vi "Relay Auto Tune.VI"(4 "calculate":bool, 5 "autotuning parameters":T3={"Controller Type"=0, "# of cycles to avg"=3, "Relay amplitude (%)"=0.0, "Control design  "=0, "Noise level %"=0.25} {"Noise level %" format="%.2f"; "Control design" items=["Normal", "Fast", "Slow"]; "Relay amplitude (%)" format="%.2f"; "Controller Type" items=["PID", "PI", "P"]}, 6 "options":T2={"sp low"=0.0, "sp high"=100.0, "out low"=-100.0, "out high"=100.0, "hold (F)"=FALSE, "auto (T)"=TRUE, "pro. band (F)"=FALSE, "reverse acting (T)"=TRUE, "beta"=1.0, "linearity"=1.0, "dt (s)"=-1.0} {"dt (s)" format="%.2f"; "linearity" min=0.0 max=1.0 format="%.2f"; "sp low" format="%.2f"; "sp high" format="%.2f"; "out low" format="%.2f"; "out high" format="%.2f"; "beta" min=0.0 max=1.0 format="%.2f"}, 7 "Prev. control out":dbl format="%.2f", 8 "Gain Scheduling Variable":dbl format="%.2f", 9 "gain scheduling":T1={"gain schedule"=[100.0], "PID parameters"=[{"Kc"=4.851751673610237, "Ti (min)"=0.021111111111111112, "Td (min)"=0.005277777777777778}], "scheduling input"=0} {"scheduling input" items=["Set-point", "Process variable", "Controller output", "Gain scheduling input"]; "PID parameters"."Td (min)" format="%.4f"; "PID parameters"."Ti (min)" format="%.4f"; "PID parameters"."Kc" format="%.4f"; "gain schedule" format="%.2f"}, 10 "PV%":dbl(slide)=19.583333333333336 scale=0.0..100.0 scale format="%.1f", 11 "setpoint (%)":dbl(slide)=30.8641975308642 scale=0.0..100.0 scale format="%.1f") -> (0 "setpoint relay":dbl(slide)=30.8641975308642 scale=0.0..100.0 scale format="%.1f", 1 "tuning status":bool, 2 "Tuned PID Parameters":T4 {"Ti" format="%.2f"; "Td" format="%.2f"})   [LabVIEW 2020, in "NI_PID__autopid compat.lvlib"]
doc: "This VI performs the setpoint relay experiment for the autotuning procedure."
uses:
  <vilib>/addons/control/pid/NI_PID__autopid compat.lvlib
  <vilib>/Analysis/baseanly.llb/Mean (DBL).vi
  <vilib>/Analysis/NI_AALBase.lvlib
panel:
  # "Relay Auto Tune"
  # "SP & PV range:"
  # "Output range:"
  # "-1: default,using\nsystem clock"
  # "Prop Band (%)"
  # "Reset Time (min)"
  # "Deriv Time (min)"
  # "Index"
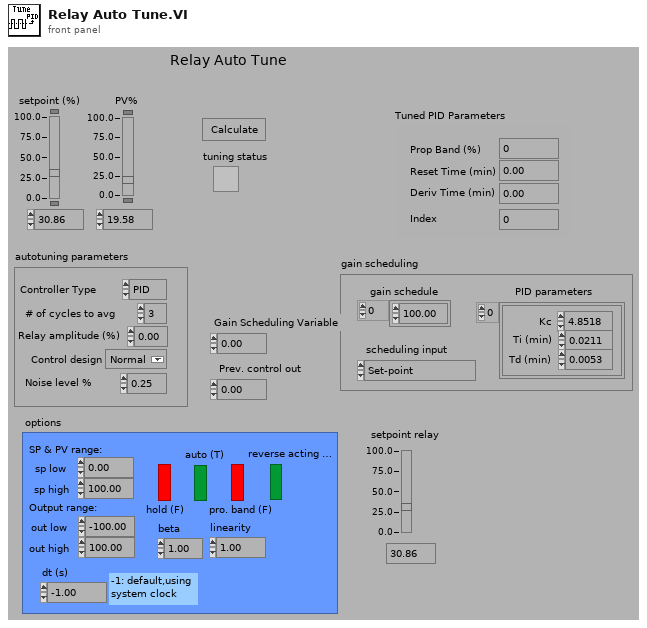
[diagram p1: front panel]
types:
  T1 = cluster{"gain schedule":dbl[], "PID parameters":cluster{"Kc":dbl, "Ti (min)":dbl, "Td (min)":dbl}[], "scheduling input":u16}
  T2 = cluster{"sp low":dbl, "sp high":dbl, "out low":dbl, "out high":dbl, "hold (F)":bool, "auto (T)":bool, "pro. band (F)":bool, "reverse acting (T)":bool, "beta":dbl, "linearity":dbl, "dt (s)":dbl}
  T3 = cluster{"Controller Type":u16, "# of cycles to avg":i32, "Relay amplitude (%)":dbl, "Control design  ":u16, "Noise level %":dbl}
  T4 = cluster{"Kc":dbl, "Ti":dbl, "Td":dbl, "Index":i32}
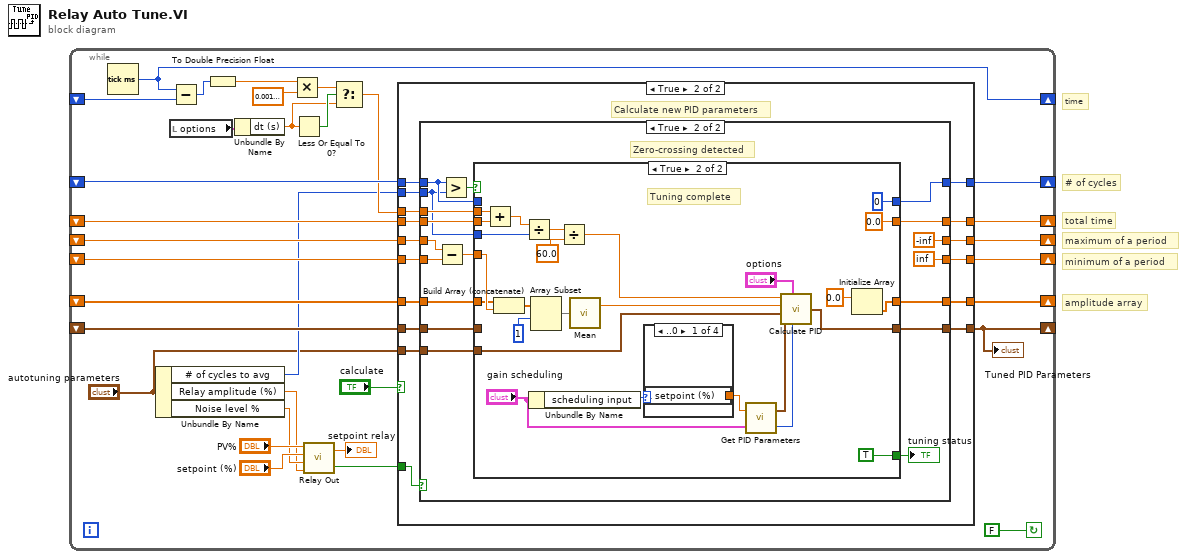
[diagram p0: block diagram]
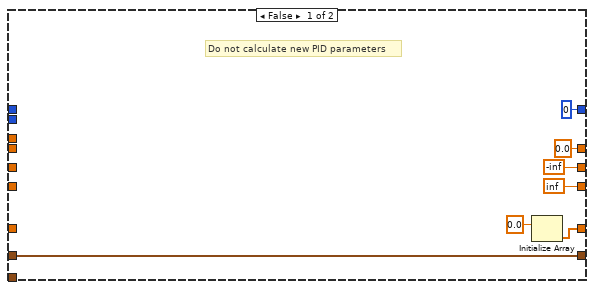
[diagram p2: hidden frame]
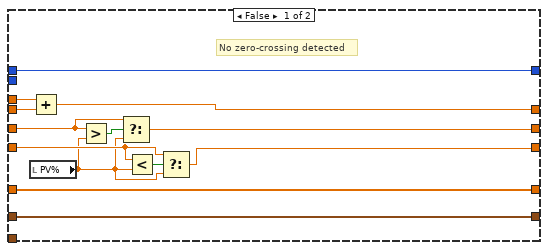
[diagram p3: hidden frame]
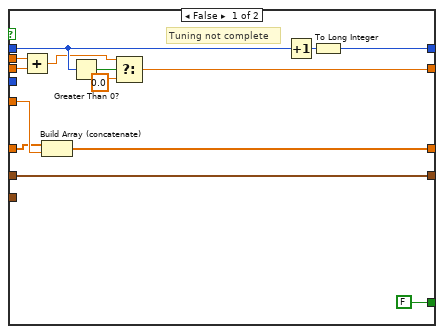
[diagram p4: hidden frame]
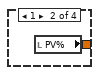
[diagram p5: hidden frame]
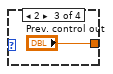
[diagram p6: hidden frame]
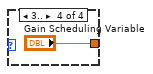
[diagram p7: hidden frame]
diagram:
  # "time"
  # "amplitude array"
  # "total time"
  # "minimum of a period"
  # "maximum of a period"
  # "# of cycles"
  n1 = while {
    shift-left: _ -> [w7]
    shift-right: [w6] -> _
    shift-left: _ -> [w12]
    shift-right: [w13] -> _
    shift-left: _ -> [w23]
    shift-right: [w20] -> _
    shift-left: _ -> [w27]
    shift-right: [w28] -> _
    shift-left: _ -> [w26]
    shift-right: [w29] -> _
    shift-left: _ -> [w30]
    shift-right: [w31] -> _
    shift-left: _ -> [w25]
    shift-right: [w32] -> _
    stop <- FALSE continue-if-true
    n2 = Tick Count (ms)() -> (millisecond timer value=w13:u32)
    n3 = Unbundle By Name("autotuning parameters") -> ("# of cycles to avg"=w3:i32, "Relay amplitude (%)"=w4:dbl, "Noise level %"=w5:dbl)
    n4 = local read "options"() -> (w10:T2)
    n5 = Subtract(x=w13, y=w12) -> (x-y=w16:u32)
    n6 = To Double Precision Float(number=w16) -> (double precision float=w17:dbl)
    n7 = Unbundle By Name(w10) -> ("dt (s)"=w14:dbl)
    n8 = Multiply(x=w17, y=0.0010000000474974513) -> (x*y=w18:dbl)
    n9 = Less Or Equal To 0?(x=w14) -> (x <= 0?=w19:bool)
    n10 = call <vilib>:"Relay Out.vi"("Relay Amp (%)"=w4, "noise disturbance %"=w5, "setpoint %"="setpoint (%)", "PV %"="PV%") -> ("Zero Crossing"=w22:bool, "relay output"=→"setpoint relay":dbl)
    n11 = Select(t=w18, s=w19, f=w14) -> (s? t:f=w11:dbl)
    n12 = case shown="True" "calculate" {
      tunnel: w25 -> [_ w43]
      tunnel: [0 w44] -> w32
      tunnel: [-inf w45] -> w31
      tunnel: w30 -> [_ w55]
      tunnel: w26 -> [_ w54]
      tunnel: [w33 w47] -> w29
      tunnel: [inf w46] -> w28
      tunnel: w27 -> [_ w48]
      tunnel: w3 -> [_ w52]
      tunnel: [w39 w49] -> w20
      tunnel: w23 -> [w39 w53]
      tunnel: w22 -> [_ w51]
      tunnel: w11 -> [_ w50]
      tunnel: w7 -> [_ w42]
      tunnel: [0.0 ("f") w41] -> w6
      tunnel: "autotuning parameters" -> [_ w40]
      frame False {
        # "Do not calculate new PID parameters"
        n13 = Initialize Array(0.0) -> (w33:dbl[])  [unwired: 1 out]
      }
      frame True {
        # "Calculate new PID parameters"
        n14 = case shown="True" w51 {
          tunnel: w43 -> [w68 w73]
          tunnel: [w68 w75] -> w44
          tunnel: [w67 -inf] -> w45
          tunnel: w55 -> [w66 w86]
          tunnel: w54 -> [w65 w84]
          tunnel: [w65 w82] -> w47
          tunnel: [w62 inf] -> w46
          tunnel: w48 -> [w63 w85]
          tunnel: w52 -> [_ w70]
          tunnel: w53 -> [w59 w81]
          tunnel: w50 -> [w57 w80]
          tunnel: [w59 w79] -> w49
          tunnel: w42 -> [w58 w72]
          tunnel: [w56 w71] -> w41
          tunnel: w40 -> [_ w69]
          frame False {
            # "No zero-crossing detected"
            n15 = local read "PV%"() -> (w60:dbl)
            n16 = Add(x=w57, y=w58) -> (x+y=w56:dbl)
            n17 = Greater?(x=w66, y=w60) -> (0:w61:bool)
            n18 = Select(t=w66, s=w61, f=w60) -> (s? t:f=w67:dbl)
            n19 = Less?(x=w63, y=w60) -> (x < y?=w64:bool)
            n20 = Select(t=w63, s=w64, f=w60) -> (s? t:f=w62:dbl)
          }
          frame True {
            # "Zero-crossing detected"
            n21 = Subtract(x=w86, y=w85) -> (x-y=w83:dbl)
            n22 = Greater?(x=w73, y=w70) -> (0:w74:bool)
            n23 = case shown="True" w74 {
              tunnel: w84 -> [w98 w112]
              tunnel: w83 -> [w99 w113]
              tunnel: [w100 w120] -> w82
              tunnel: [w95 0] -> w75
              tunnel: w73 -> [w92 _]
              tunnel: [FALSE TRUE] -> w78
              tunnel: [w97 w101] -> w79
              tunnel: w81 -> [w97 _]
              tunnel: w80 -> [w94 w117]
              tunnel: w72 -> [w93 w118]
              tunnel: [w88 0.0 ("f")] -> w71
              tunnel: w70 -> [_ w115]
              tunnel: w69 -> [_ w104]
              frame False {
                # "Tuning not complete"
                n24 = Add(x=w94, y=w93) -> (x+y=w90:dbl)
                n25 = Build Array (concatenate)(w98, w99) -> (w100:dbl[])
                n26 = Greater Than 0?(x=w92) -> (x > 0?=w91:bool)
                n27 = Select(t=w90, s=w91, f=0.0) -> (s? t:f=w88:dbl)
                n28 = Increment(x=w92) -> (x+1=w96:i32)
                n29 = To Long Integer(number=w96) -> (32bit integer=w95:i32)
              }
              frame True {
                # "Tuning complete"
                n30 = Add(x=w117, y=w118) -> (x+y=w116:dbl)
                n31 = Build Array (concatenate)(w112, w113) -> (w111:dbl[])
                n32 = Divide(x=w116, y=w115) -> (x/y=w114:dbl)
                n33 = Unbundle By Name("gain scheduling") -> ("scheduling input"=w108:u16)
                n34 = Array Subset(array=w111, index=1) -> (w123:dbl[])  [unwired: 1 in]
                n35 = Divide(x=w114, y=60.0) -> (x/y=w103:dbl)
                n36 = call-poly <vilib>:"Mean.vi"("X"=w123) -> ("mean"=w105:dbl)  [unwired: 1 out]
                n37 = case shown="..0" w108 {
                  tunnel: [w127 w128 "Prev. control out" "Gain Scheduling Variable"] -> w109
                  frame ..0 {
                    n38 = local read "setpoint (%)"() -> (w127:dbl)
                  }
                  frame 1 {
                    n39 = local read "PV%"() -> (w128:dbl)
                  }
                  frame 2 {
                  }
                  frame 3.. {
                  }
                }
                n40 = call <vilib>:"Get PID Parameters.vi"("gain scheduling"="gain scheduling", "scheduling variable"=w109) -> ("scheduling index"=w106:i32, "PID parameters"=w107:cluster{"Kp":dbl, "Ti":dbl, "Td":dbl})
                n41 = call <vilib>:"Calculate PID.vi"("scheduling index"=w106, "options"="options", "PID parameters"=w107, "autotuning parameters"=w104, "Mean amplitude"=w105, "Mean period"=w103) -> ("Tuned PID Parameters"=w101:T4)
                n42 = Initialize Array(0.0) -> (w120:dbl[])  [unwired: 1 out]
              }
            }
            "tuning status" <- w78
          }
        }
      }
    }
    "Tuned PID Parameters" <- w20
  }
